vi "ClearLastLF.vi"(11 "spreadsheet string in":string) -> (3 "spreadsheet string out":string)   [LabVIEW 2016]
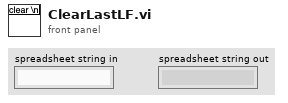
[diagram p1: front panel]
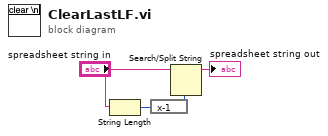
[diagram p0: block diagram]
diagram:
  n1 = String Length(string="spreadsheet string in") -> (length=w3:i32)
  n2 = expression code="x-1"(w3) -> (w4:i32)
  n3 = Search/Split String(string="spreadsheet string in", offset (0)=w4) -> (substring before match=→"spreadsheet string out":string)  [unwired: 1 in, 2 out]
